vi "UDP Data Link - Configuration Utilities - Initialize Main Page Panel.vi"(8 "error in (no error)":errorcluster, 10 "Main Page References":T1, 11 "Item Ref in":T2 format="%.0x") -> (0 "error out":errorcluster, 3 "Item Ref out":T2 format="%.0x")   [LabVIEW 2015, in "UDP-Custom-Device System Explorer.lvlib"]
doc: "Initializes the Main Page front panel from the properties."
uses:
  UDP-Custom-Device System Explorer.lvlib
  <vilib>/NI Veristand/Custom Device API/Custom Device Item Ref.ctl
  Types/UDP Data Link - TypeDefs - Main Page References.ctl
  Shared/Constants.vi
  <vilib>/NI Veristand/Custom Device API/Get Item Property (I32).vi
  <vilib>/NI Veristand/Custom Device API/Get Item Property (Boolean).vi
  <vilib>/NI Veristand/Custom Device API/Get Item Property (String).vi
  <vilib>/NI Veristand/Custom Device API/Set Item Property (String).vi
  <vilib>/NI Veristand/Custom Device API/Get Item Property (U16).vi
  <vilib>/NI Veristand/Custom Device API/Get Item Property (Dependent Node Pointer).vi
  <vilib>/NI VeriStand/Custom Device API/Custom Device API.lvlib
  Shared/UDP-Custom-Device Shared.lvlib
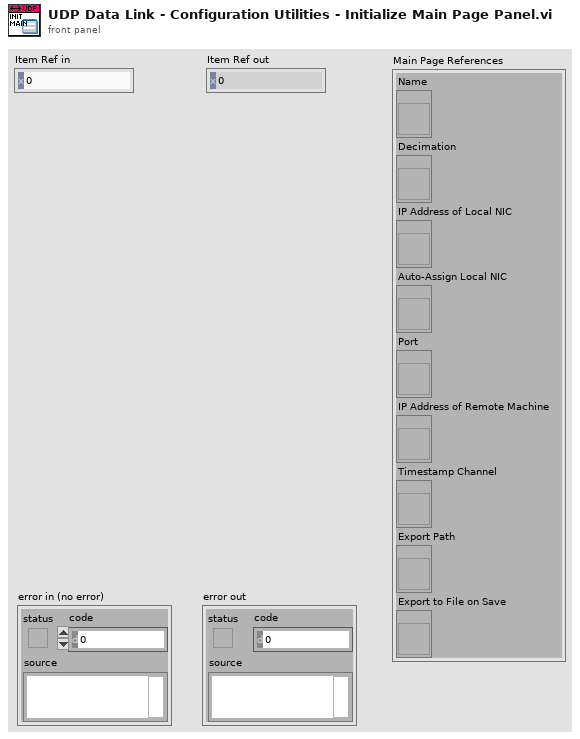
[diagram p1: front panel]
types:
  T1 = typedef "UDP-Custom-Device System Explorer.lvlib/UDP Data Link - TypeDefs - Main Page References.ctl" = cluster{"Name":refnum<vi>, "Decimation":refnum<vi>, "IP Address of Local NIC":refnum<vi>, "Auto-Assign Local NIC":refnum<vi>, "Port":refnum<vi>, "IP Address of Remote Machine":refnum<vi>, "Timestamp Channel":refnum<vi>, "Export Path":refnum<vi>, "Export to File on Save":refnum<vi>}
  T2 = typedef "Custom Device API.lvlib/Custom Device Item Ref.ctl" = u64
  T3 = typedef "Custom Device API.lvlib/Custom Device Item Info.ctl" = cluster{"Name":string, "Is Channel":bool, "GUID":string, "Is Waveform":bool}
  T4 = enum8{"Enabled", "Disabled", "Disabled and Grayed Out"}
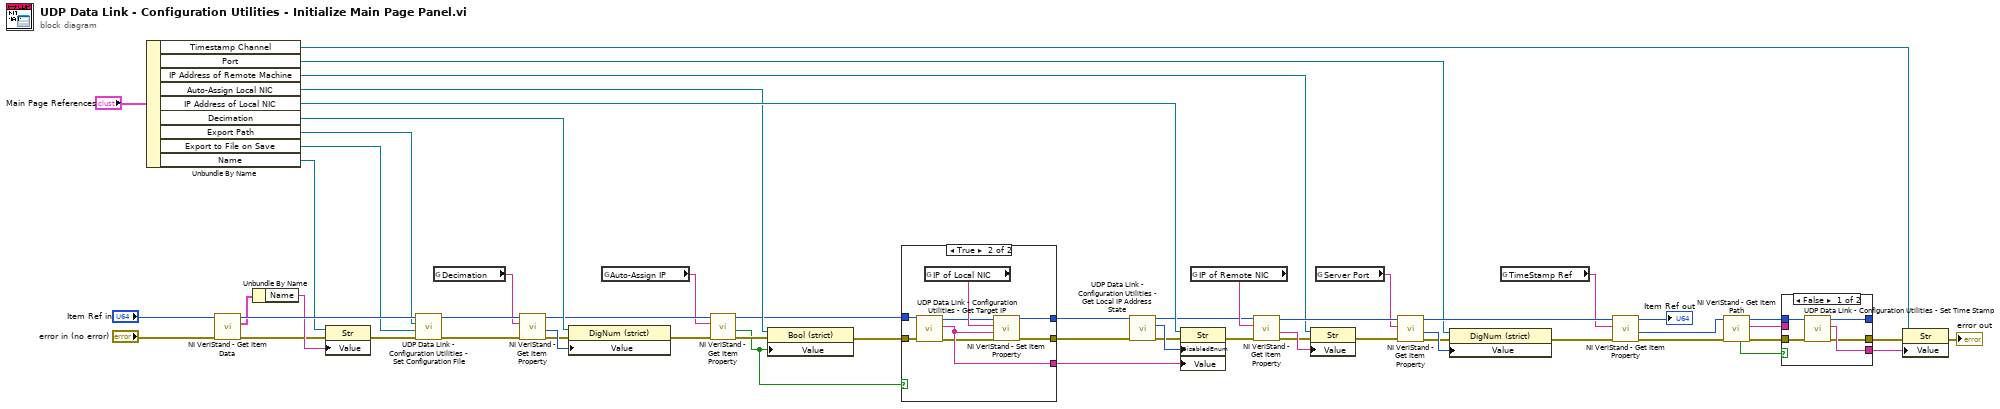
[diagram p0: block diagram]
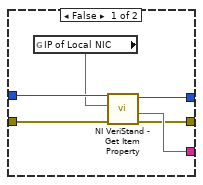
[diagram p2: hidden frame]
diagram:
  n1 = Unbundle By Name("Main Page References") -> ("Timestamp Channel"=w19:refnum<vi>, "Port"=w20:refnum<vi>, "IP Address of Remote Machine"=w23:refnum<vi>, "Auto-Assign Local NIC"=w28:refnum<vi>, "IP Address of Local NIC"=w29:refnum<vi>, "Decimation"=w30:refnum<vi>, "Export Path"=w32:refnum<vi>, "Export to File on Save"=w33:refnum<vi>, "Name"=w36:refnum<vi>)
  n2 = call <vilib>:"NI VeriStand - Get Item Data.vi"("error in (no error)"="error in (no error)", "Item Ref in"="Item Ref in") -> ("error out"=w35:errorcluster, "Item Info"=w38:T3, "Item Ref out"=w57:T2)  [unwired: 7 out]
  n3 = Unbundle By Name(w38) -> ("Name"=w39:string)
  n4 = property class="Str"(reference=w36, error in=w35, "Value"=w39) -> (error out=w34:errorcluster)  [unwired: 1 out]
  n5 = call "UDP Data Link - Configuration Utilities - Set Configuration File.vi"("error in (no error)"=w34, "Export to File on Save"=w33, "Export Path"=w32, "Item Ref in"=w57) -> ("error out"=w56:errorcluster, "Item Ref out"=w55:T2)  [unwired: 6 in]
  n6 = global read "Constants.vi" "Decimation"() -> (w1:string)
  n7 = call-poly <vilib>:"NI VeriStand - Get Item Property.vi"("error in (no error)"=w56, "Property Name"=w1, "Item Ref in"=w55) -> ("error out"=w31:errorcluster, "Value"=w54:i32, "Item Ref out"=w15:T2)  [unwired: 5 in, 1 out]
  n8 = property class="DigNum (strict)"(reference=w30, error in=w31, "Value"=w54) -> (error out=w16:errorcluster)  [unwired: 1 out]
  n9 = global read "Constants.vi" "Auto-Assign IP"() -> (w2:string)
  n10 = call-poly <vilib>:"NI VeriStand - Get Item Property.vi"("error in (no error)"=w16, "Property Name"=w2, "Item Ref in"=w15) -> ("error out"=w27:errorcluster, "Value"=w11:bool, "Item Ref out"=w13:T2)  [unwired: 5 in, 1 out]
  n11 = property class="Bool (strict)"(reference=w28, error in=w27, "Value"=w11) -> (error out=w14:errorcluster)  [unwired: 1 out]
  n12 = case shown="True" w11 {
    tunnel: [w63 w65] -> w26
    tunnel: [w62 w71] -> w6
    tunnel: [w61 w70] -> w7
    tunnel: w14 -> [w60 w67]
    tunnel: w13 -> [w59 w66]
    frame False {
      n13 = global read "Constants.vi" "IP of Local NIC"() -> (w58:string)
      n14 = call-poly <vilib>:"NI VeriStand - Get Item Property.vi"("error in (no error)"=w60, "Property Name"=w58, "Item Ref in"=w59) -> ("error out"=w62:errorcluster, "Value"=w63:string, "Item Ref out"=w61:T2)  [unwired: 5 in, 1 out]
    }
    frame True {
      n15 = call "UDP Data Link - Configuration Utilities - Get Target IP.vi"("error in"=w67, "Item Ref in"=w66) -> ("error out"=w64:errorcluster, "IPAddress"=w65:string, "Item Ref out"=w68:T2)  [unwired: 7 in]
      n16 = global read "Constants.vi" "IP of Local NIC"() -> (w69:string)
      n17 = call-poly <vilib>:"NI VeriStand - Set Item Property.vi"("error in (no error)"=w64, "Value"=w65, "Property Name"=w69, "Item Ref in"=w68) -> ("error out"=w71:errorcluster, "Item Ref out"=w70:T2)  [unwired: 5 in, 1 out]
    }
  }
  n18 = call "UDP Data Link - Configuration Utilities - Get Local IP Address State.vi"("error in (no error)"=w6, "Item Ref in"=w7) -> ("error out"=w3:errorcluster, "State"=w4:T4, "Item Ref out"=w5:T2)  [unwired: 7 in]
  n19 = property on="Property Node" class="Str"(reference=w29, error in=w3, "DisabledEnum"=w4, "Value"=w26) -> (error out=w12:errorcluster)  [unwired: 1 out]
  n20 = global read "Constants.vi" "IP of Remote NIC"() -> (w8:string)
  n21 = call-poly <vilib>:"NI VeriStand - Get Item Property.vi"("error in (no error)"=w12, "Property Name"=w8, "Item Ref in"=w5) -> ("error out"=w25:errorcluster, "Value"=w42:string, "Item Ref out"=w43:T2)  [unwired: 5 in, 1 out]
  n22 = property class="Str"(reference=w23, error in=w25, "Value"=w42) -> (error out=w24:errorcluster)  [unwired: 1 out]
  n23 = global read "Constants.vi" "Server Port"() -> (w10:string)
  n24 = call-poly <vilib>:"NI VeriStand - Get Item Property.vi"("error in (no error)"=w24, "Property Name"=w10, "Item Ref in"=w43) -> ("error out"=w22:errorcluster, "Value"=w44:u16, "Item Ref out"=w45:T2)  [unwired: 5 in, 1 out]
  n25 = property class="DigNum (strict)"(reference=w20, error in=w22, "Value"=w44) -> (error out=w21:errorcluster)  [unwired: 1 out]
  n26 = global read "Constants.vi" "TimeStamp Ref"() -> (w9:string)
  n27 = call-poly <vilib>:"NI VeriStand - Get Item Property.vi"("error in (no error)"=w21, "Property Name"=w9, "Item Ref in"=w45) -> ("error out"=w47:errorcluster, "Dependent Node Ref"=w53:T2, "Item Ref out"=→"Item Ref out":T2)  [unwired: 5 in, 1 out]
  n28 = call <vilib>:"NI VeriStand - Get Item Path.vi"("error in (no error)"=w47, "Item Ref in"=w53) -> ("error out"=w51:errorcluster, "Path"=w49:string, "Item Ref out"=w50:T2, "Found"=w48:bool)  [unwired: 6 in]
  n29 = case shown="False" w48 {
    tunnel: w49 -> [_ w78]
    tunnel: w50 -> [w75 w79]
    tunnel: w51 -> [w76 w77]
    tunnel: [w74 w79] -> _
    tunnel: [w73 w78] -> w52
    tunnel: [w72 w77] -> w18
    frame False {
      n30 = call "UDP Data Link - Configuration Utilities - Set Time Stamp.vi"("error in (no error)"=w76, "Device Item Ref in"=w75) -> ("error out"=w72:errorcluster, "Path"=w73:string, "Device Item Ref out"=w74:T2)  [unwired: 7 in]
    }
    frame True {
    }
  }
  n31 = property class="Str"(reference=w19, error in=w18, "Value"=w52) -> (error out=→"error out":errorcluster)  [unwired: 1 out]
